vi "Dereferncing 1D Array Pointer Long.vi"(8 "error in (no error)":errorcluster, 10 "1D Double Array Pointer":u64, 11 "numberOfSamples":u32) -> (0 "error out":errorcluster, 3 "Array Data":i32[](array[numeric]))   [LabVIEW 2022 SP3, in "MU_3SL_interface.lvlib"]
uses:
  MU_3SL_interface.lvlib
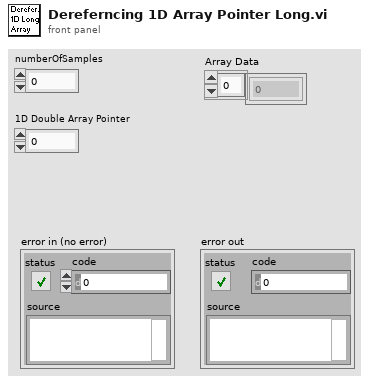
[diagram p1: front panel]
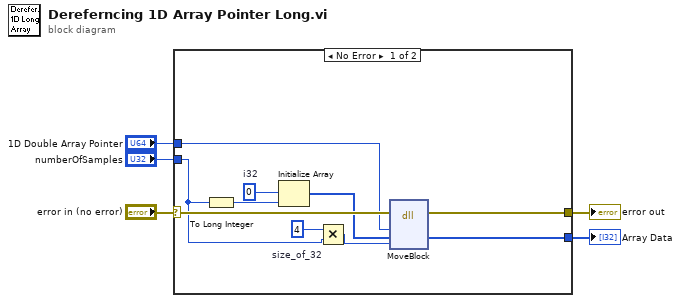
[diagram p0: block diagram]
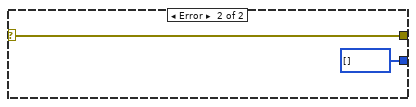
[diagram p2: hidden frame]
diagram:
  n1 = case shown="No Error" "error in (no error)" {
    selector: "error in (no error)" -> [w15 w17]
    tunnel: "numberOfSamples" -> [w7 _]
    tunnel: "1D Double Array Pointer" -> [w11 _]
    tunnel: [w8 w17] -> w4
    tunnel: [w14 i32[] [] ("dest")] -> w3
    frame No Error {
      w10 = u32 4  # size_of_32
      w12 = 0  # i32
      n2 = To Long Integer(number=w7) -> (32bit integer=w6:i32)
      n3 = Initialize Array(w12, w6) -> (w13:i32[])
      n4 = Multiply(x=w10, y=w7) -> (x*y=w9:u32)
      n5 = dll-call lib="LabVIEW" fn="MoveBlock"(error in=w15, "source"=w11, "dest"=w13, "size"=w9) -> (error out=w8:errorcluster, "dest"=w14:i32[])  [unwired: 5 in, 1 out]
    }
    frame Error {
    }
  }
  "error out" <- w4
  "Array Data" <- w3
